vi "publishSummaryState.vi"(8 "error in (no error)":errorcluster, 11 "SummaryState":i32) -> (0 "error out":errorcluster)   [LabVIEW 2016]
uses:
  SALLV_Test/DataTypes/logevent_summaryState.ctl
  SALLV_Test/SALLV_Test.lvlib
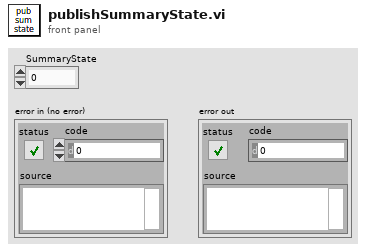
[diagram p1: front panel]
types:
  T1 = typedef "SALLV_Test.lvlib/logevent_summaryState.ctl" = cluster{"summaryState":i32, "priority":i32}
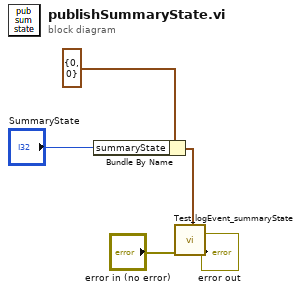
[diagram p0: block diagram]
diagram:
  n1 = Bundle By Name(cluster=T1 {"summaryState"=0, "priority"=0} ("logevent_summaryState_Ctl"), "summaryState"="SummaryState") -> (w4:T1)
  n2 = call "Test_logEvent_summaryState.vi"("error in (no error)"="error in (no error)", "logevent_summaryState_Ctl"=w4) -> ("error out"=→"error out":errorcluster)  [unwired: 7 in, 2 out]
